vi "Rotate Tile.vi"(8 "error in (no error)":errorcluster, 9 "Target":i32, 10 "Current":i32, 11 "Tile in":refnum<class "Tile.lvclass">) -> (0 "error out":errorcluster, 3 "Tile out":refnum<class "Tile.lvclass">)   [LabVIEW 2020, in "Tile.lvclass"]
uses:
  Tile.lvclass
  Tile.lvclass/Tile.ctl
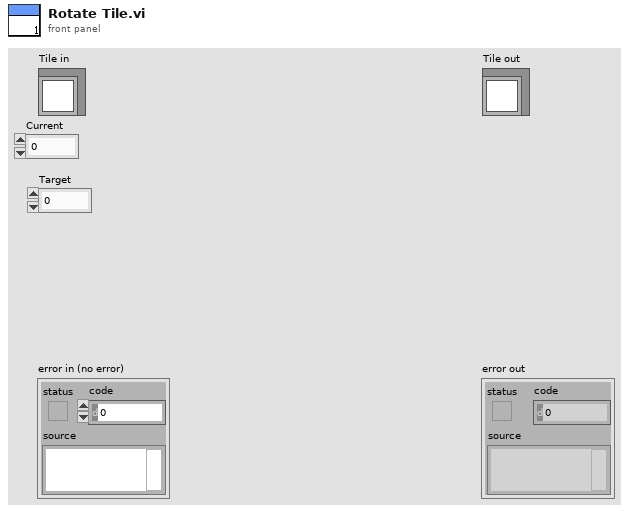
[diagram p1: front panel]
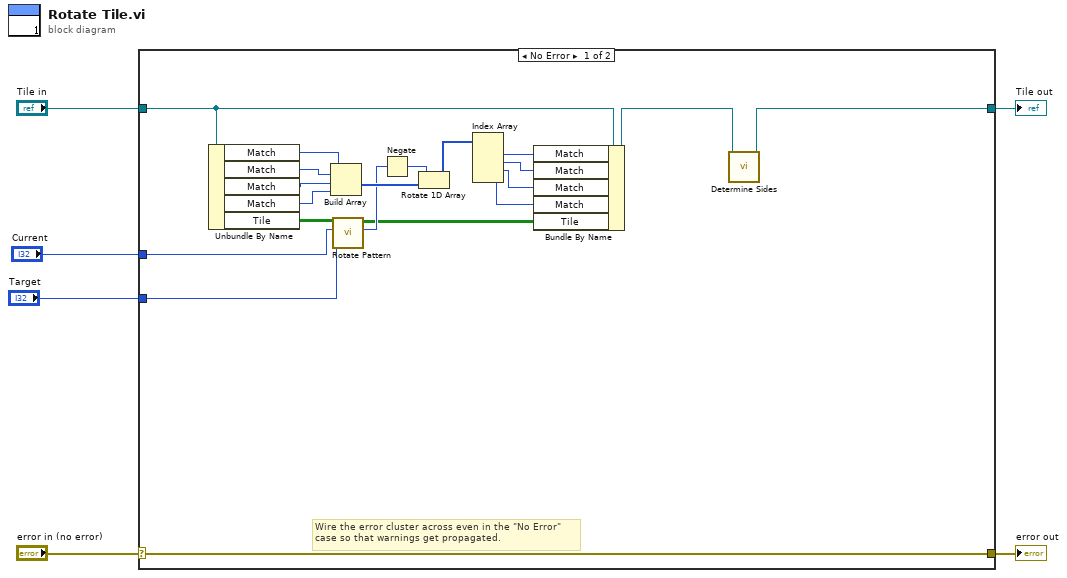
[diagram p0: block diagram]
diagram:
  n1 = case shown="No Error" "error in (no error)" {
    selector: "error in (no error)" -> [w26 w28]
    tunnel: [w26 w28] -> w5
    tunnel: [w7 w27] -> w3
    tunnel: "Tile in" -> [w24 w27]
    tunnel: "Current" -> [w10 _]
    tunnel: "Target" -> [w9 _]
    frame No Error {
      # "Wire the error cluster across even in the \"No Error\"\ncase so that warnings get propagated."
      n2 = Unbundle By Name(w24) -> ("Match"=w20:u64, "Match"=w21:u64, "Match"=w22:u64, "Match"=w23:u64, "Tile"=w25:bool[][])
      n3 = Build Array(w20, w21, w22, w23) -> (w19:u64[])
      n4 = call "Rotate Pattern.vi"("Target"=w9, "Current"=w10, "Pattern In"=w25) -> ("Rotation CCW"=w18:i32, "Pattern Out"=w16:bool[][])  [unwired: 7 in]
      n5 = Negate(x=w18) -> (-x=w17:i32)
      n6 = Rotate 1D Array(1:w19, 2:w17) -> (0:w15:u64[])
      n7 = Index Array(array=w15) -> (element #1=w14:u64, element #2=w11:u64, element #3=w12:u64, element #4=w13:u64)  [unwired: 4 in]
      n8 = Bundle By Name(cluster=w24, "Match"=w14, "Match"=w11, "Match"=w12, "Match"=w13, "Tile"=w16) -> (w8:refnum<class "Tile.lvclass">)
      n9 = call "Determine Sides.vi"("Tile in"=w8) -> ("Tile out"=w7:refnum<class "Tile.lvclass">)  [unwired: 9 in, 1 out]
    }
    frame Error {
    }
  }
  "error out" <- w5
  "Tile out" <- w3
